vi "MainProcess.vi"(8 "error in (no error)":errorcluster, 9 "System Status Ref.":refnum<vi>, 10 "pound in":refnum<class "Pound.lvclass">, 11 "qbus in":refnum<class "Qbus.lvclass">) -> (0 "error out":errorcluster, 2 "Pound":refnum<class "Pound.lvclass">, 3 "Qbus out":refnum<class "Qbus.lvclass">)   [LabVIEW 2015, in "System.lvlib"]
uses:
  System.lvlib
  <vilib>/addons/Qbus/Qbus.lvclass
  <vilib>/NI/Software Watchdog/Pound/Pound.lvclass
  FileHandler/FileHandler.lvlib
  <vilib>/addons/TimerProcess/TimerProcess.lvlib
  MainController/MainController.lvlib
  CopyUtility/CopyUtility.lvlib
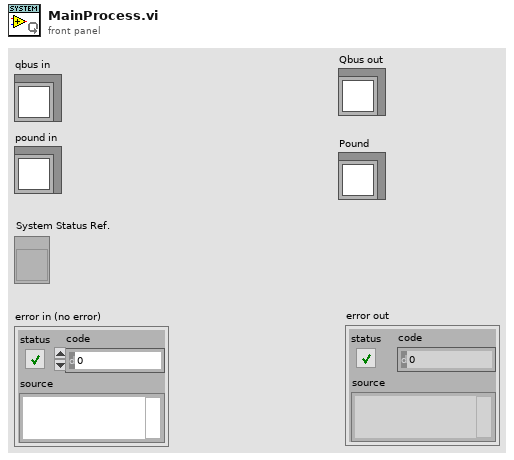
[diagram p1: front panel]
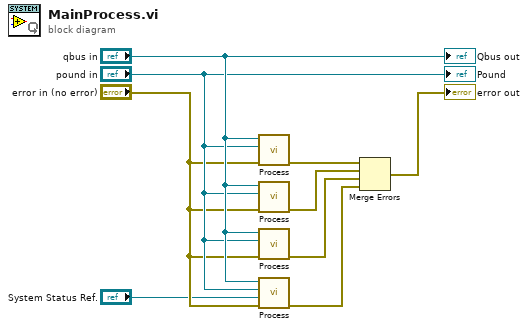
[diagram p0: block diagram]
diagram:
  n1 = call <vilib>:"Process.vi"("error in (no error)"="error in (no error)", "pound in"="pound in", "qbus in"="qbus in") -> ("error out"=w9:errorcluster)  [unwired: 8 in]
  n2 = call <vilib>:"Process.vi"("error in (no error)"="error in (no error)", "pound in"="pound in", "qbus in"="qbus in") -> ("error out"=w8:errorcluster)  [unwired: 8 in]
  n3 = call <vilib>:"Process.vi"("error in (no error)"="error in (no error)", "pound in"="pound in", "qbus in"="qbus in") -> ("error out"=w7:errorcluster)  [unwired: 8 in]
  n4 = call <vilib>:"Process.vi"("error in (no error)"="error in (no error)", "System Status Ref."="System Status Ref.", "pound in"="pound in", "qbus in"="qbus in") -> ("error out"=w5:errorcluster)  [unwired: 7 in]
  n5 = Merge Errors(w9, w8, w7, w5) -> (→"error out":errorcluster)
  "Qbus out" <- "qbus in"
  "Pound" <- "pound in"
